vi "AFM_Driver_Manager.InitializeDrivers.vi"(8 "error in (no error)":errorcluster, 10 "Paths":path[](array[path]), 11 "AFM_Driver_Manager in":refnum<class "AFM_Driver_Manager.lvclass">) -> (0 "error out":errorcluster, 3 "AFM_Driver_Manager out":refnum<class "AFM_Driver_Manager.lvclass">)   [LabVIEW 2019, in "AFM_Driver_Manager.lvclass"]
doc: "Takes a list of paths to Drivers, programmatically start them, create API's using events, and populate their front panel controls with the correct values needed for further communication."
uses:
  AFM_Driver_Manager.lvclass
  AFM_Driver_Manager.lvclass/AFM_Driver_Manager.ctl
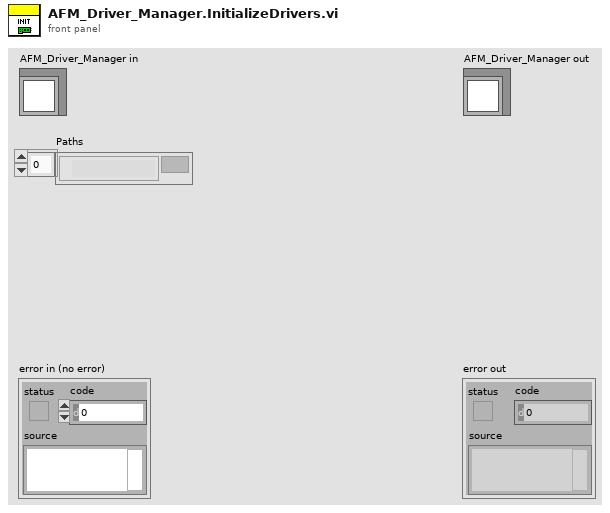
[diagram p1: front panel]
types:
  T1 = typedef "AFM_Driver_Manager.lvclass/AFM_Driver_Manager.PublicMethods.ctl" = cluster{"Stop Event":refnum<user-event>, "Lithography Data":refnum<user-event>, "Run Lithography":refnum<user-event>, "Background Image":refnum<user-event>, "Abort Notifier":refnum<user-event>}
  T2 = cluster{"VI Refnum":refnum<vi>, "Path":path, "Name":string, "Events":T1}[]
  T3 = typedef "AFM_Driver_Manager.lvclass/AFM_Driver_Manager.PublicEvents.ctl" = cluster{"Lithography Done":refnum<user-event>}
  T4 = cluster{"VI Refnum":refnum<vi>, "Path":path, "Name":string, "Events":T1}
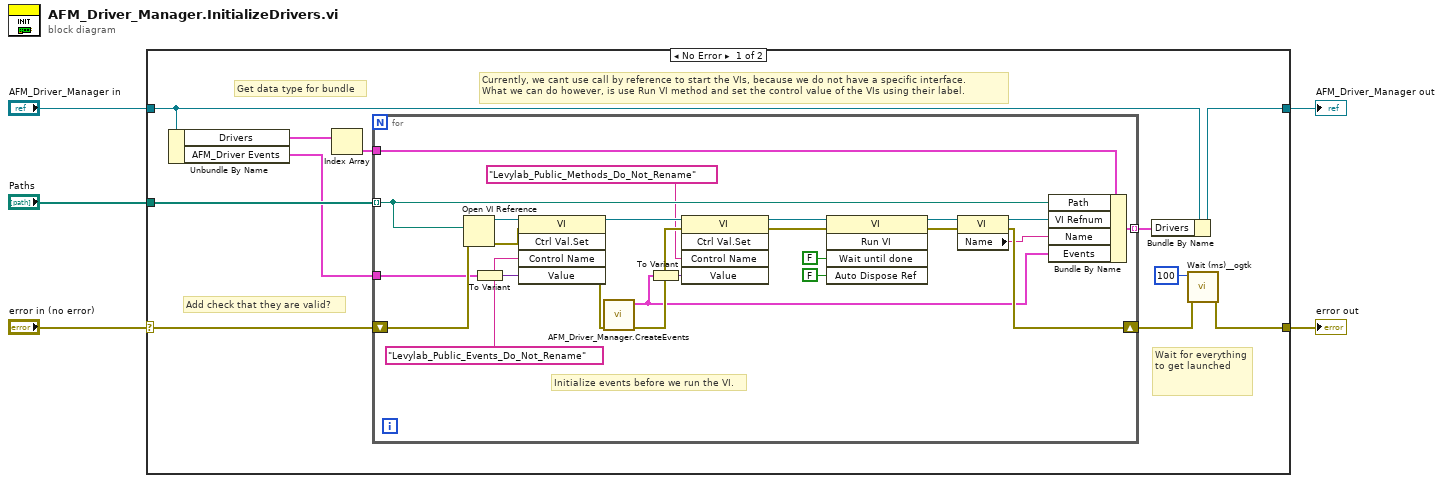
[diagram p0: block diagram]
diagram:
  n1 = case shown="No Error" "error in (no error)" {
    selector: "error in (no error)" -> [w10 w42]
    tunnel: [w7 w42] -> w4
    tunnel: [w15 w41] -> w2
    tunnel: "AFM_Driver_Manager in" -> [w14 w41]
    tunnel: "Paths" -> [w16 _]
    frame No Error {
      # "Wait for everything to get launched"
      # "Get data type for bundle"
      # "Add check that they are valid?"
      # "Currently, we cant use call by reference to start the VIs, because we do not have a specific interface.\nWhat we can do however, is use Run VI method and set the control value of the VIs using their label."
      n2 = Unbundle By Name(w14) -> ("Drivers"=w12:T2, "AFM_Driver Events"=w9:T3)
      n3 = Index Array(array=w12) -> (element=w11:T4)  [unwired: 1 in]
      n4 = for {
        tunnel: w16 -> [w30] mode=indexing
        shift-right: [w37] -> w8
        shift-left: w10 -> [w39]
        tunnel: w11 -> [w32]
        tunnel: [w28] -> w13 mode=indexing
        tunnel: w9 -> [w20]
        # "Initialize events before we run the VI."
        n5 = Open VI Reference(vi path=w30, error in (no error)=w39) -> (vi reference=w27:refnum<vi>, error out=w25:errorcluster)  [unwired: 4 in]
        n6 = To Variant(anything=w20) -> (Variant=w21:variant)
        n7 = invoke on="Invoke Node" class="VI" method="Ctrl Val.Set"(reference=w27, error in=w25, "Control Name"="Levylab_Public_Events_Do_Not_Rename", "Value"=w21) -> (reference out=w26:refnum<vi>, error out=w17:errorcluster)  [unwired: 1 in, 3 out]
        n8 = call "AFM_Driver_Manager.CreateEvents.vi"("error in (no error)"=w17) -> ("error out"=w24:errorcluster, "Events Cluster"=w18:T1)  [unwired: 9 in]
        n9 = To Variant(anything=w18) -> (Variant=w19:variant)
        n10 = invoke on="Invoke Node" class="VI" method="Ctrl Val.Set"(reference=w26, error in=w24, "Control Name"="Levylab_Public_Methods_Do_Not_Rename", "Value"=w19) -> (reference out=w34:refnum<vi>, error out=w40:errorcluster)  [unwired: 1 in, 3 out]
        n11 = invoke on="Invoke Node" class="VI" method="Run VI"(reference=w34, error in=w40, "Wait until done"=FALSE ("Wait Until Done"), "Auto Dispose Ref"=FALSE ("Auto Dispose Reference")) -> (reference out=w33:refnum<vi>, error out=w38:errorcluster)  [unwired: 1 in, 3 out]
        n12 = property on="Property Node" class="VI"(reference=w33, error in=w38) -> (reference out=w31:refnum<vi>, error out=w37:errorcluster, "Name"=w29:string)
        n13 = Bundle By Name(cluster=w32, "Path"=w30, "VI Refnum"=w31, "Name"=w29, "Events"=w18) -> (w28:T4)
      }
      n14 = Bundle By Name(cluster=w14, "Drivers"=w13) -> (w15:refnum<class "AFM_Driver_Manager.lvclass">)
      n15 = call <userlib>:"Wait (ms)__ogtk.vi"("error in (no error)"=w8, "milliseconds to wait"=u32 100) -> ("error out"=w7:errorcluster)  [unwired: 8 in, 1 out]
    }
    frame Error {
    }
  }
  "error out" <- w4
  "AFM_Driver_Manager out" <- w2
